vi "IIR DAQ Filter.vi"() -> ()   [LabVIEW 2009]
uses:
  <vilib>/DAQmx/configure/timing.llb/DAQmx Timing (Sample Clock).vi
  <vilib>/DAQmx/create/channels.llb/DAQmx Create Channel (AI-Voltage-Basic).vi
  Instance          11 22Saved   IIR DAQ Filter .vi
  <vilib>/DAQmx/read.llb/DAQmx Read (Analog Wfm 1Chan NSamp).vi
  <vilib>/express/express analysis/Spectral/XNode/ExpressSpectralMeasurementsBlockNode.xnode
  <vilib>/express/express analysis/Spectral/Block/exnSpectralBlock spectral measurements power poly.vi
  <vilib>/express/express analysis/Spectral/Block/exnSpectralBlock spectral measurements power DDT.vi
panel:
  out "Filtered Frequency Domain":dynamicdata(graph)
  out "Prefiltered Frequency Domain":dynamicdata(graph)
  in  "stop":bool
  out "Filtered Time Domain":dynamicdata(graph) caption="Filtered Signal"
  out "Prefiltered Time Domain":waveform(dbl)(graph)
  in  "samples per channel":i32=1000
  in  "rate":dbl=1000.0 format="%0.2f"
  in  "physical channels":tag
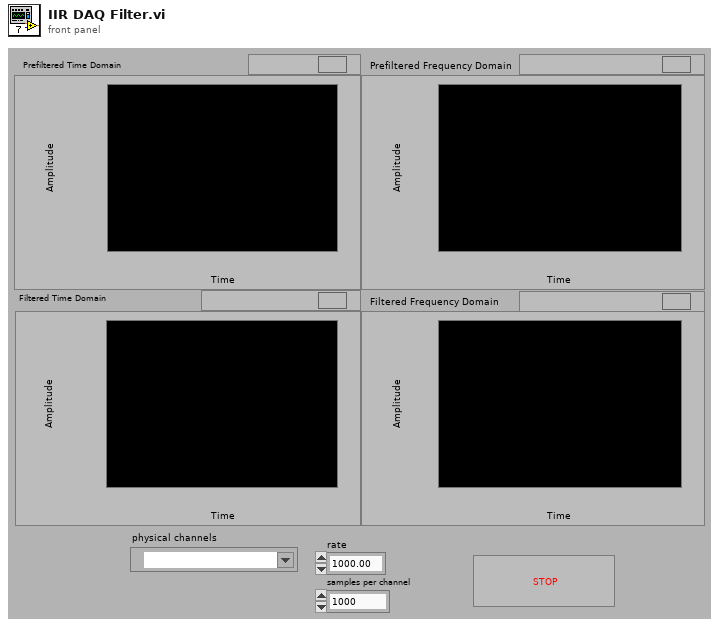
[diagram p1: front panel]
types:
  T1 = cluster{"averaging mode":u16, "weighting mode":u16, "number of averages":u32}
  T2 = cluster{"dB On (F)":bool, "unwrap phase (F)":bool, "convert to degree (F)":bool}
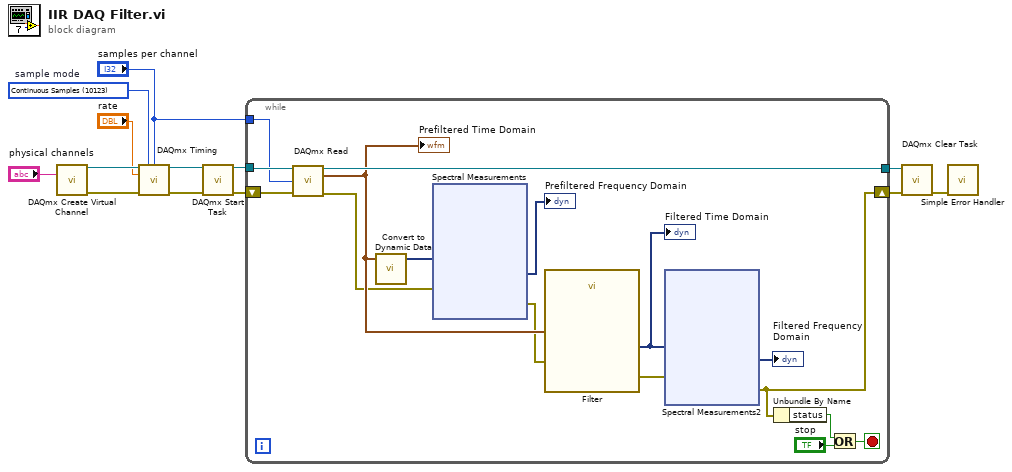
[diagram p0: block diagram]
diagram:
  w9 = 10123 items=["Finite Samples"=10178, "Continuous Samples"=10123]  # sample mode
  n1 = call-poly <vilib>:"DAQmx Create Virtual Channel.vi"("physical channels"="physical channels") -> ("task out"=w12:refnum<k21>, "error out"=w11:errorcluster)  [unwired: 13 in]
  n2 = call-poly <vilib>:"DAQmx Timing.vi"("task/channels in"=w12, "sample mode"=w9, "samples per channel"="samples per channel", "rate"="rate", "error in"=w11) -> ("task out"=w8:refnum<k21>, "error out"=w7:errorcluster)  [unwired: 9 in]
  n3 = call <vilib>:"DAQmx Start Task.vi"("task/channels in"=w8, "error in"=w7) -> ("task out"=w6:refnum<k21>, "error out"=w5:errorcluster)  [unwired: 12 in]
  n4 = while {
    tunnel: w6 -> [w29]
    tunnel: [w27] -> w4
    tunnel: "samples per channel" -> [w17]
    shift-right: [w22] -> w2
    shift-left: w5 -> [w28]
    stop <- w24 stop-if-true
    n5 = call-poly <vilib>:"DAQmx Read.vi"("task/channels in"=w29, "number of samples per channel"=w17, "error in"=w28) -> ("task out"=w27:refnum<k21>, "data"=w26:waveform(dbl), "error out"=w15:errorcluster)  [unwired: 10 in]
    "Prefiltered Time Domain" <- w26
    n6 = call "Convert to Dynamic Data"("Waveform"=w26) -> ("Dynamic Data Type"=w16:dynamicdata)  [unwired: 3 in]
    n7 = xnode "Spectral Measurements"("Signals"=w16, "error in (no error)"=w15) -> ("Power Spectrum"=→"Prefiltered Frequency Domain":dynamicdata, "error out"=w21:errorcluster)
    n8 = call "Filter"("error in (no error)"=w21, "Signal"=w26) -> ("error out"=w20:errorcluster, "Filtered Signal"=w19:dynamicdata)  [unwired: 8 in]
    "Filtered Time Domain" <- w19
    n9 = xnode "Spectral Measurements2"("Signals"=w19, "error in (no error)"=w20) -> ("Power Spectrum"=→"Filtered Frequency Domain":dynamicdata, "error out"=w22:errorcluster)
    n10 = Unbundle By Name "Unbundle By Name"(w22) -> ("status"=w18:bool)
    n11 = Or(x=w18, y="stop") -> (x .or. y?=w24:bool)
  }
  n12 = call <vilib>:"DAQmx Clear Task.vi"("task in"=w4, "error in"=w2) -> ("error out"=w3:errorcluster)  [unwired: 13 in]
  n13 = call <vilib>:"Simple Error Handler.vi"("error in (no error)"=w3) -> ()  [unwired: 4 in, 5 out]
